vi "Get Status.vi"(8 "error in (no error)":errorcluster, 11 "Motor in":refnum<class "Motor.lvclass">) -> (0 "error out":errorcluster, 3 "Motor out":refnum<class "Motor.lvclass">)   [LabVIEW 2019, in "Motor.lvclass"]
uses:
  Motor.lvclass
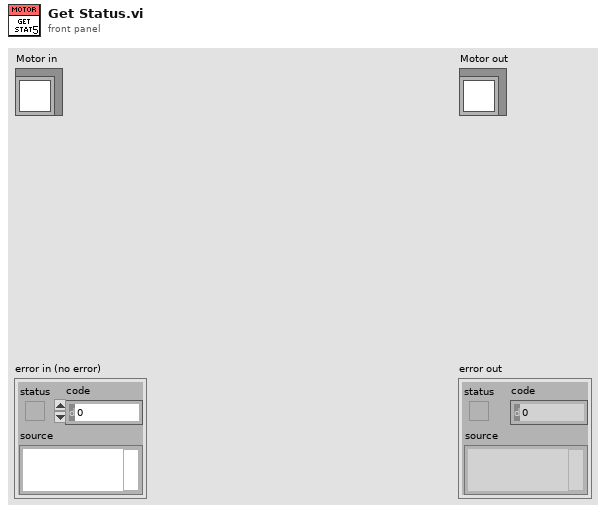
[diagram p1: front panel]
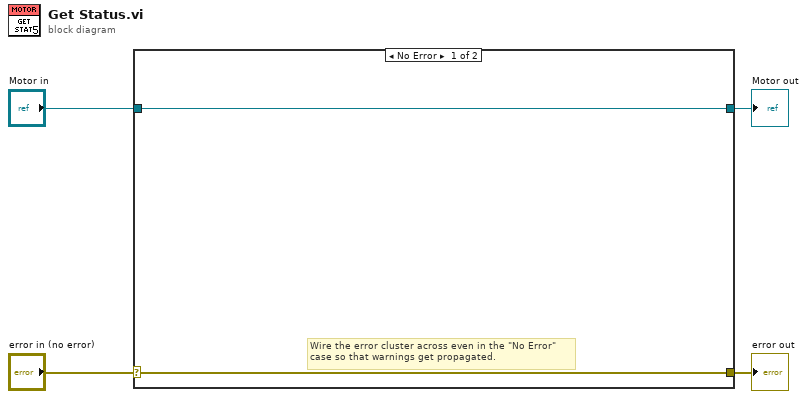
[diagram p0: block diagram]
diagram:
  n1 = case shown="No Error" "error in (no error)" {
    selector: "error in (no error)" -> [w5 w8]
    tunnel: [w5 w8] -> w3
    tunnel: [w6 w7] -> w1
    tunnel: "Motor in" -> [w6 w7]
    frame No Error {
      # "Wire the error cluster across even in the \"No Error\"\ncase so that warnings get propagated."
    }
    frame Error {
    }
  }
  "error out" <- w3
  "Motor out" <- w1
